vi "niScope Multi Fetch Measurement Stats.vi"(0 "instrument handle":refnum<k15>, 1 "timeout":dbl=5.0 format="%.2f", 5 "channels":string="0", 7 "scalar measurement":T1=4000 items=["None"=4000, "Frequency"=2, "Average Frequency"=1016, "FFT Frequency"=1008, "Period"=3, "Average Period"=1015, "Rise Time"=0, "Fall Time"=1, "Rising Slew Rate"=1010, "Falling Slew Rate"=1011, "Overshoot"=18, "Preshoot"=19, "Voltage RMS"=4, "Voltage Cycle RMS"=16, "AC Estimate"=1012, "FFT Amplitude"=1009, "Voltage Average"=10, "Voltage Cycle Average"=17, "DC Estimate"=1013, "Voltage Max"=6, "Voltage Min"=7, "Voltage Peak-to-Peak"=5, "Voltage High"=8, "Voltage Low"=9, "Voltage Amplitude"=15, "Voltage Top"=1007, "Voltage Base"=1006, "Voltage Base-to-Top"=1017, "Negative Width"=11, "Positive Width"=12, "Negative Duty Cycle"=13, "Positive Duty Cycle"=14, "Integral"=1005, "Area"=1003, "Cycle Area"=1004, "Time Delay"=1014, "Phase Delay"=1018, "Low Ref Volts"=1000, "Mid Ref Volts"=1001, "High Ref Volts"=1002, "Volt. Hist. Mean"=2000, "Volt. Hist. Stdev"=2001, "Volt. Hist. Median"=2003, "Volt. Hist. Mode"=2010, "Volt. Hist. Max"=2005, "Volt. Hist. Min"=2006, "Volt. Hist. Peak-to-Peak"=2002, "Volt. Hist. Mean + Stdev"=2007, "Volt. Hist. Mean + 2 Stdev"=2008, "Volt. Hist. Mean + 3 Stdev"=2009, "Volt. Hist. Hits"=2004, "Volt. Hist. New Hits"=2011, "Time Hist. Mean"=3000, "Time Hist. Stdev"=3001, "Time Hist. Median"=3003, "Time Hist. Mode"=3010, "Time Hist. Max"=3005, "Time Hist. Min"=3006, "Time Hist. Peak-to-Peak"=3002, "Time Hist. Mean + Stdev"=3007, "Time Hist. Mean + 2 Stdev"=3008, "Time Hist. Mean + 3 Stdev"=3009, "Time Hist. Hits"=3004, "Time Hist. New Hits"=3011], 11 "error in":errorcluster) -> (4 "instrument handle out":refnum<k15>, 6 "stats":T2(array[cluster]) {"max" format="%^.2e"; "min" format="%^.2e"; "stdev" format="%^.2e"; "mean" format="%^.2e"; "scalar result" format="%^.2e"}, 15 "error out":errorcluster)   [LabVIEW 2011]
doc: "Obtains a waveform measurement and returns the measurement value for multiple channel and multiple record acquisitions."
uses:
  <instrlib>/niScope/Controls/niScope scalar measurement.ctl
  niScope_32.dll
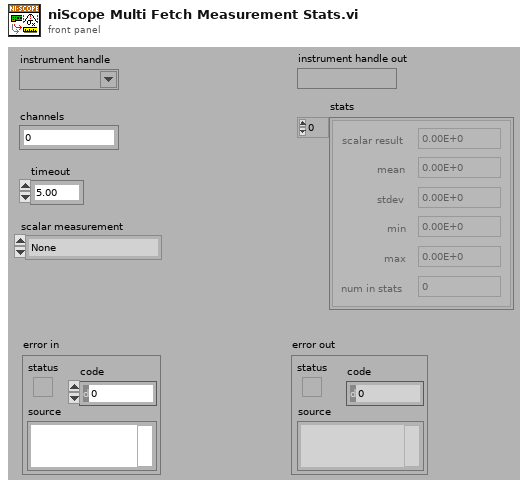
[diagram p1: front panel]
types:
  T1 = typedef "niScope scalar measurement.ctl" = i32
  T2 = cluster{"scalar result":dbl, "mean":dbl, "stdev":dbl, "min":dbl, "max":dbl, "num in stats":i32}[]
  T3 = cluster{"scalar result":dbl, "mean":dbl, "stdev":dbl, "min":dbl, "max":dbl, "num in stats":i32}
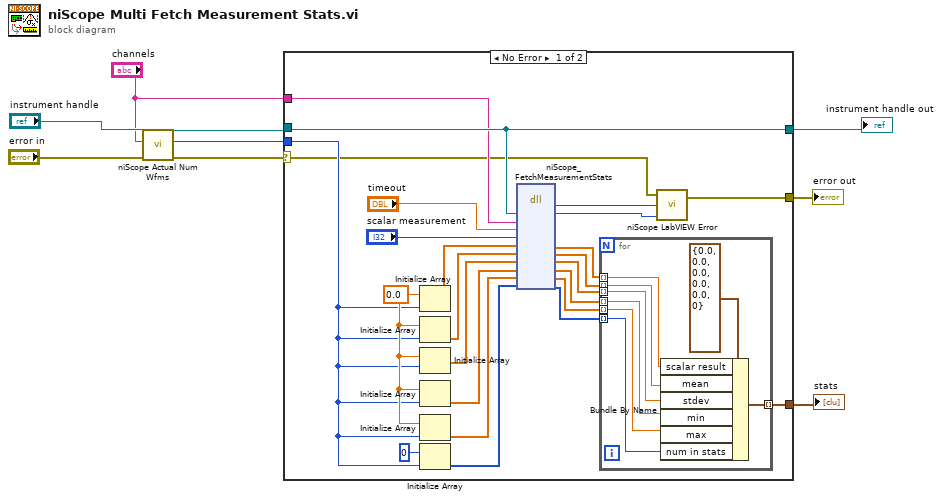
[diagram p0: block diagram]
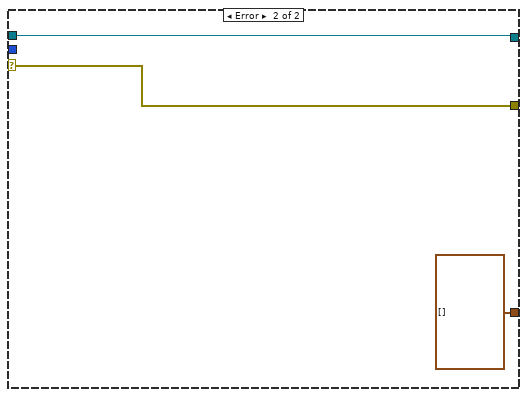
[diagram p2: hidden frame]
diagram:
  n1 = call <instrlib>:"niScope Actual Num Wfms.vi"("error in"="error in", "channels"="channels", "instrument handle"="instrument handle") -> ("error out"=w1:errorcluster, "actual num wfms"=w2:i32, "instrument handle out"=w6:refnum<k15>)  [unwired: 6 in]
  n2 = case shown="No Error" w1 {
    selector: w1 -> [w10 w42]
    tunnel: [w33 w42] -> w9
    tunnel: w6 -> [w28 w43]
    tunnel: [w29 T2 []] -> w8
    tunnel: [w28 w43] -> w7
    tunnel: "channels" -> [w26 _]
    tunnel: w2 -> [w25 _]
    frame No Error {
      w27 = 0.0 ("Element Data")
      n3 = Initialize Array(w27, w25) -> (w19:dbl[])
      n4 = Initialize Array(w27, w25) -> (w20:dbl[])
      n5 = Initialize Array(w27, w25) -> (w21:dbl[])
      n6 = Initialize Array(w27, w25) -> (w22:dbl[])
      n7 = Initialize Array(w27, w25) -> (w23:dbl[])
      n8 = Initialize Array(0 ("Element Data"), w25) -> (w24:i32[])
      n9 = dll-call lib="niScope_*.*" fn="niScope_FetchMeasurementStats"("instrument handle"=w28, "channelList"=w26, "timeout"="timeout", "scalarMeasFunction"="scalar measurement", "results"=w19, "means"=w20, "stdevs"=w21, "mins"=w22, "maxs"=w23, "numInStats"=w24) -> ("status"=w32:i32, "instrument handle"=w31:u32, "results"=w11:dbl[], "means"=w12:dbl[], "stdevs"=w13:dbl[], "mins"=w14:dbl[], "maxs"=w15:dbl[], "numInStats"=w16:i32[])  [unwired: 6 in, 2 out]
      n10 = for {
        tunnel: w11 -> [w40] mode=indexing
        tunnel: w12 -> [w39] mode=indexing
        tunnel: w13 -> [w38] mode=indexing
        tunnel: w14 -> [w37] mode=indexing
        tunnel: w15 -> [w36] mode=indexing
        tunnel: w16 -> [w35] mode=indexing
        tunnel: [w34] -> w29 mode=indexing
        n11 = Bundle By Name(cluster=T3 {"scalar result"=0.0, "mean"=0.0, "stdev"=0.0, "min"=0.0, "max"=0.0, "num in stats"=0} ("First Measurement"), "scalar result"=w40, "mean"=w39, "stdev"=w38, "min"=w37, "max"=w36, "num in stats"=w35) -> (w34:T3)
      }
      n12 = call <instrlib>:"niScope LabVIEW Error.vi"("instrument handle"=w31, "niScope error code (0)"=w32, "error in (no error)"=w10) -> ("error out"=w33:errorcluster)  [unwired: 2 in]
    }
    frame Error {
    }
  }
  "instrument handle out" <- w7
  "error out" <- w9
  "stats" <- w8
